vi "add delta delay(SubVI).vi"(10 "字符串":string) -> (1 "ok or cancel":bool, 2 "连接的字符串":string)   [LabVIEW 2019, in "Add Seq.lvlib"]
uses:
  Add Seq.lvlib
panel:
  in  "delta delay time":dbl
  in  "cancel":bool
  in  "ok":bool
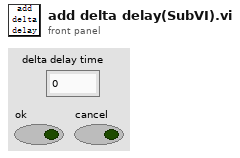
[diagram p1: front panel]
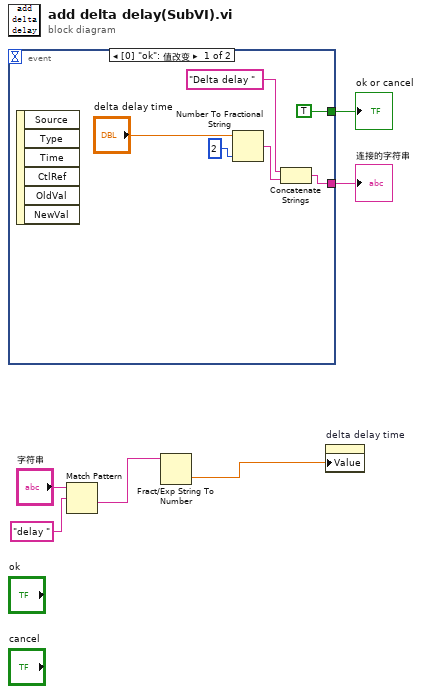
[diagram p0: block diagram]
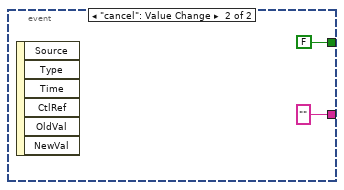
[diagram p2: hidden frame]
diagram:
  n1 = event shown="[0] \"ok\": 值改变" {
    selector: _ -> [_ _]
    dyn-events: _ -> [_ _]
    timeout: _ -> [_ _]
    tunnel: [TRUE FALSE] -> w6
    tunnel: [w7 "" ("分隔符")] -> w5
    event "ok": Value Change {
      n2 = event-data() -> ()  [unwired: 1 in, 6 out]
      n3 = Number To Fractional String(number="delta delay time", precision (6)=i16 2 ("精度(6)")) -> (F-format string=w9:string)  [unwired: 2 in]
      n4 = Concatenate Strings("Delta delay " ("字符串"), w9) -> (w7:string)
    }
    event "cancel": Value Change {
      n5 = event-data() -> ()  [unwired: 1 in, 6 out]
    }
  }
  "ok or cancel" <- w6
  "连接的字符串" <- w5
  n6 = Match Pattern(string="字符串", regular expression="delay " ("正则表达式")) -> (after substring=w3:string)  [unwired: 1 in, 3 out]
  n7 = Fract/Exp String To Number(string=w3) -> (number=w2:dbl)  [unwired: 3 in, 1 out]
  n8 = property on="delta delay time" class="DigNum (严格)"("Value"=w2) -> ()  [unwired: 2 in, 2 out]
